vi "Time_FGV_실습.vi"() -> ()   [LabVIEW 2020]
panel:
  out "경과시간 2":dbl
  out "경과시간":dbl
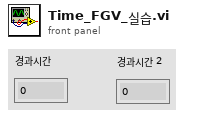
[diagram p1: front panel]
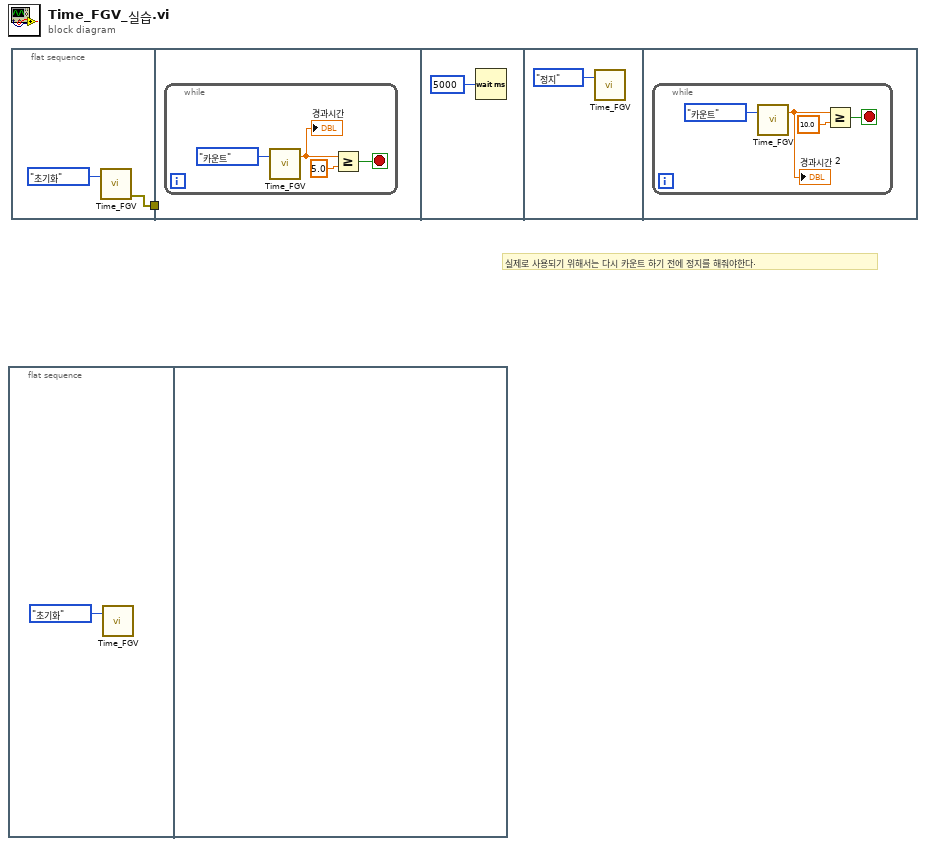
[diagram p0: block diagram]
diagram:
  # "실제로 사용되기 위해서는 다시 카운트 하기 전에 정지를 해줘야한다."
  n1 = flat-sequence {
    frame #0 {
      n2 = call "Time_FGV.vi"("상태"=enum16{"초기화", "카운트", "정지"}."초기화") -> ()  [unwired: 1 in, 2 out]
    }
    frame #1 {
    }
  }
  n3 = flat-sequence {
    tunnel: [w3] -> w1
    tunnel: w1 -> [_]
    frame #0 {
      n4 = call "Time_FGV.vi"("상태"=enum16{"초기화", "카운트", "정지"}."초기화") -> ("에러 상수 2"=w3:errorcluster)  [unwired: 1 in, 1 out]
    }
    frame #1 {
      n5 = while {
        stop <- w5 stop-if-true
        n6 = call "Time_FGV.vi"("상태"=enum16{"초기화", "카운트", "정지"}."카운트") -> ("경과시간"=w7:dbl)  [unwired: 1 in, 1 out]
        "경과시간" <- w7
        n7 = Greater Or Equal?(x=w7, y=5.0) -> (x >= y?=w5:bool)
      }
    }
    frame #2 {
      n8 = Wait (ms)(milliseconds to wait=u32 5000 ("대기 시간 (ms)")) -> ()  [unwired: 1 out]
    }
    frame #3 {
      n9 = call "Time_FGV.vi"("상태"=enum16{"초기화", "카운트", "정지"}."정지") -> ()  [unwired: 1 in, 2 out]
    }
    frame #4 {
      n10 = while {
        stop <- w11 stop-if-true
        n11 = call "Time_FGV.vi"("상태"=enum16{"초기화", "카운트", "정지"}."카운트") -> ("경과시간"=w13:dbl)  [unwired: 1 in, 1 out]
        "경과시간 2" <- w13
        n12 = Greater Or Equal?(x=w13, y=10.0) -> (x >= y?=w11:bool)
      }
    }
  }
